vi "Stand Alone Temp.vi"() -> ()   [LabVIEW 2009, in "Temperature Controller.lvclass"]
uses:
  Temperature Controller.lvclass
  Global/Sound Files.vi
  Utility Classes/Instrument/Instrument.lvclass
panel:
  in  "warnON":bool caption="Warn On"
  in  "greater":bool caption="Temp Greater?"
  in  "warn":dbl caption="Warn at"
  out "nv%":dbl(slide) caption="NV" scale=0.0..100.0
  out "heater%":dbl(slide) caption="Heater" scale=0.0..100.0
  out "active":bool
  out "ok":bool
  in  "exit":bool
  out "temp":dbl
  # "On"
  # "K"
  # "K"
  # "Status"
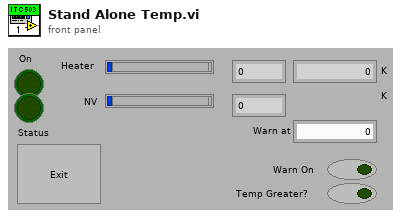
[diagram p1: front panel]
types:
  T1 = typedef "Temperature Controller.lvclass/HV Slide Indicator.ctl" = dbl
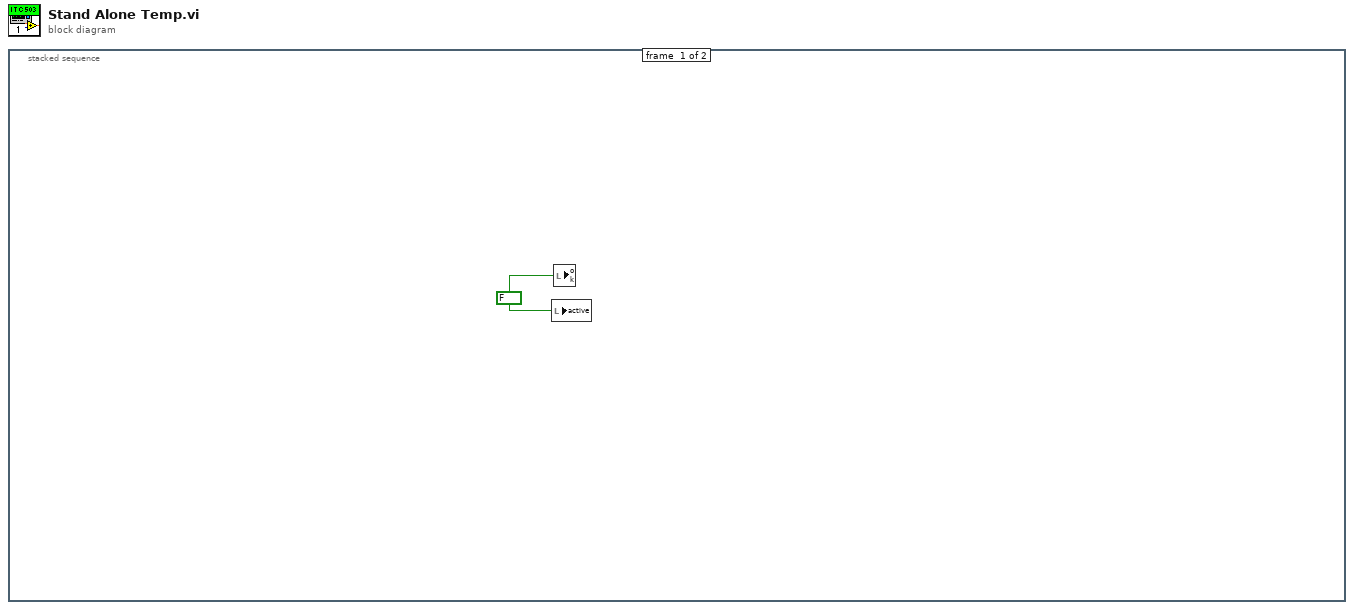
[diagram p0: block diagram]
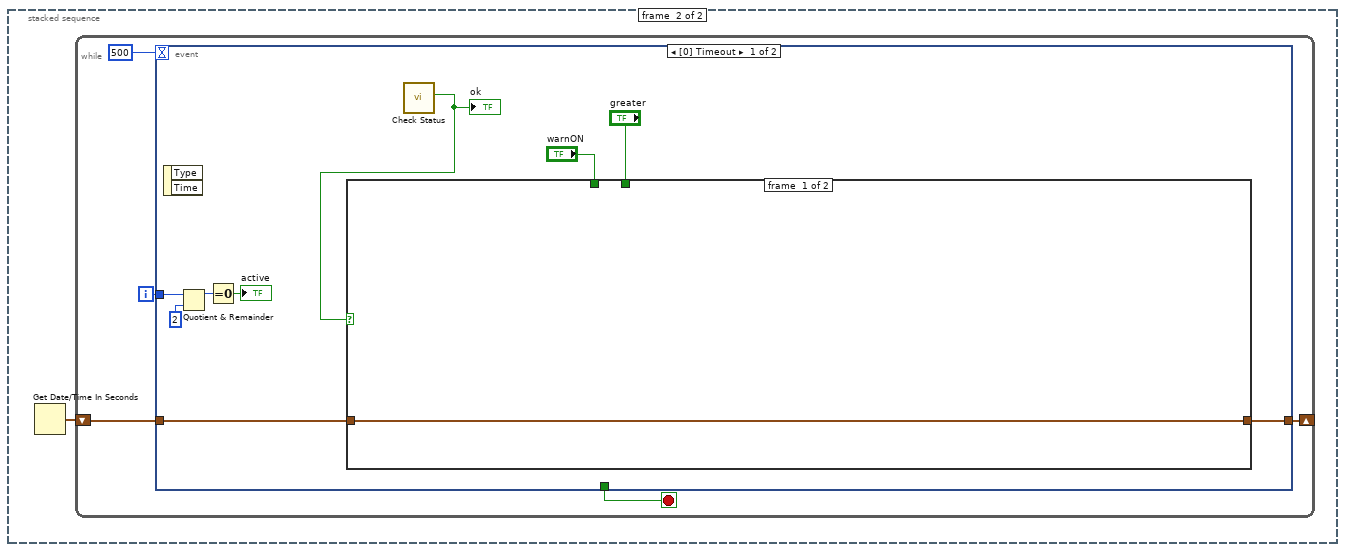
[diagram p2: hidden frame]
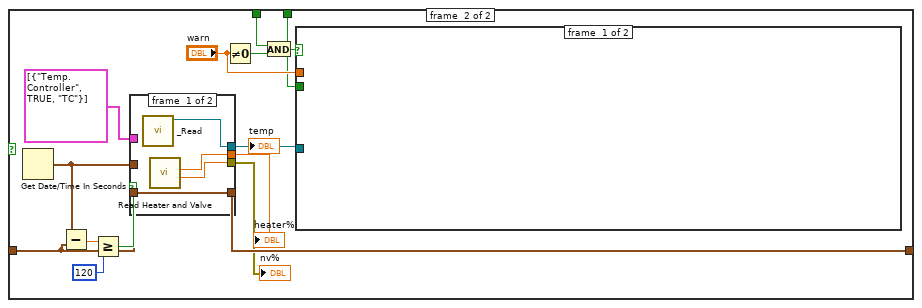
[diagram p3: hidden frame]
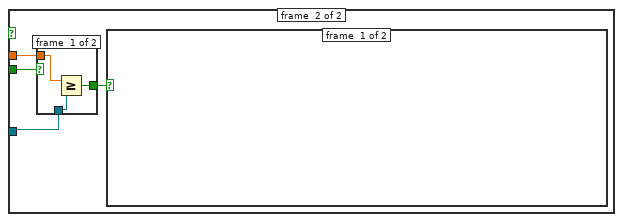
[diagram p4: hidden frame]
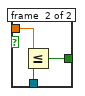
[diagram p5: hidden frame]
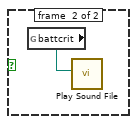
[diagram p6: hidden frame]
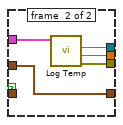
[diagram p7: hidden frame]
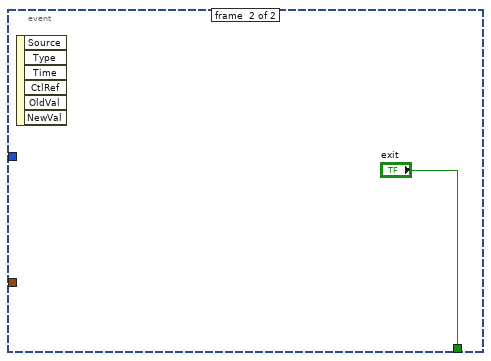
[diagram p8: hidden frame]
diagram:
  n1 = stacked-sequence {
    frame #0 {
      w1 = FALSE
      n2 = local write "active"(w1) -> ()
      n3 = local write "ok"(w1) -> ()
    }
    frame #1 {
      n4 = Get Date/Time In Seconds() -> (seconds since 1Jan1904=w2:timestamp)
      n5 = while {
        shift-right: [w3] -> _
        shift-left: w2 -> [w4]
        i -> [w5]
        stop <- w7 stop-if-true
        n6 = event shown="[0] Timeout" {
          selector: _ -> [_ _]
          dyn-events: _ -> [_ _]
          timeout: 500 -> [_ _]
          tunnel: [_ "exit"] -> w7
          tunnel: w5 -> [w16 _]
          tunnel: w4 -> [w12 _]
          tunnel: [w11 _] -> w3
          event #0 {
            n7 = event-data() -> ()  [unwired: 3 out]
            n8 = Quotient & Remainder(x=w16, y=2) -> (x-y*floor(x/y)=w14:i32)  [unwired: 1 out]
            n9 = Equal To 0?(x=w14) -> (x = 0?=→"active":bool)
            n10 = call-dynamic "Check Status.vi"() -> ("Ready?"=w8:bool)  [unwired: 8 in, 3 out]
            "ok" <- w8
            n11 = case shown="True" w8 {
              tunnel: w12 -> [w17 w27]
              tunnel: [w17 w26] -> w11
              tunnel: "greater" -> [_ w21]
              tunnel: "warnON" -> [_ w18]
              frame #0 {
              }
              frame #1 {
                n12 = Get Date/Time In Seconds() -> (seconds since 1Jan1904=w28:timestamp)
                n13 = Subtract(x=w28, y=w27) -> (x-y=w32:dbl)
                n14 = Greater Or Equal?(x=w32, y=120) -> (x >= y?=w30:bool)
                n15 = case shown="False" w30 {
                  tunnel: [w47 w52] -> w22
                  tunnel: cluster{string, bool, string}[] [{"Temp. Controller", TRUE, "TC"}] -> [_ w51]
                  tunnel: w28 -> [_ w50]
                  tunnel: w27 -> [w46 _]
                  tunnel: [w46 w50] -> w26
                  tunnel: [w44 w49] -> w25
                  tunnel: [w45 w48] -> w24
                  frame #0 {
                    n16 = call-dynamic "_Read.vi"() -> ("Temperature Controller out"=w47:refnum<class "Temperature Controller.lvclass">)  [unwired: 9 in, 2 out]
                    n17 = call-dynamic "Read Heater and Valve.vi"() -> ("valve%"=w45:T1, "heater%"=w44:T1)  [unwired: 8 in, 2 out]
                  }
                  frame #1 {
                    n18 = call-dynamic "Log Temp.vi"("Temperature Controller in"=w51) -> ("error out"=w48:errorcluster, 1:w49, 2:w52)  [unwired: 7 in, 1 out]
                  }
                }
                "temp" <- w22
                "heater%" <- w25
                "nv%" <- w24
                n19 = Not Equal To 0?(x="warn") -> (x != 0?=w19:bool)
                n20 = And(x=w18, y=w19) -> (x .and. y?=w20:bool)
                n21 = case shown="True" w20 {
                  tunnel: "warn" -> [_ w36]
                  tunnel: w22 -> [_ w35]
                  tunnel: w21 -> [_ w33]
                  frame #0 {
                  }
                  frame #1 {
                    n22 = case shown="True" w33 {
                      tunnel: w36 -> [w37 w42]
                      tunnel: w35 -> [w38 w41]
                      tunnel: [w39 w40] -> w34
                      frame #0 {
                        n23 = Greater Or Equal?(x=w37, y=w38) -> (x >= y?=w39:bool)
                      }
                      frame #1 {
                        n24 = Less Or Equal?(x=w42, y=w41) -> (x <= y?=w40:bool)
                      }
                    }
                    n25 = case shown="True" w34 {
                      frame #0 {
                      }
                      frame #1 {
                        n26 = global read "Sound Files.vi" "battcrit"() -> (w43:path)
                        n27 = call <vilib>:"Play Sound File.vi"("path"=w43) -> ()  [unwired: 3 in, 8 out]
                      }
                    }
                  }
                }
              }
            }
          }
          event #1 {
            n28 = event-data() -> ()  [unwired: 7 out]
          }
        }
      }
    }
  }
